vi "GetDeviceTransactions.vi"() -> ()   [LabVIEW 2014]
uses:
  USBAnalyzerEllisysDll/Debug/USBAnalyzerEllisysDll.dll
panel:
  out "Dev":i32[](array[numeric])
  out "devices 2":i32[](array[numeric])
  out "transactions":u64[](array[numeric])
  out "size":i32
  out "Percent %":dbl[](array[numeric]) format="%.2f"
  out "Pie Chart":picture
  out "Colors 2":u32[](array[colorbox])=[11796480, 37103, 40712, 16770816, 11796658, 4210752]
  in  "Colors":u32[](array[colorbox])=[11796480, 37103, 40712, 16770816, 11796658, 4210752]
  out "return type":i32
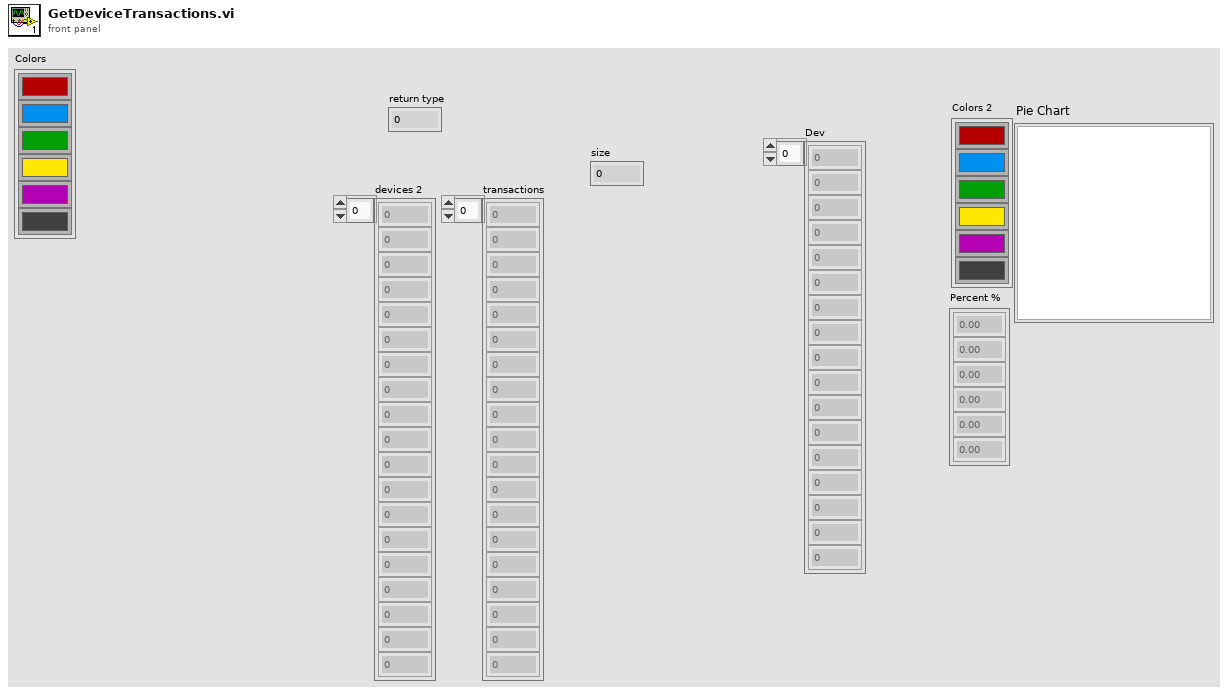
[diagram p1: front panel]
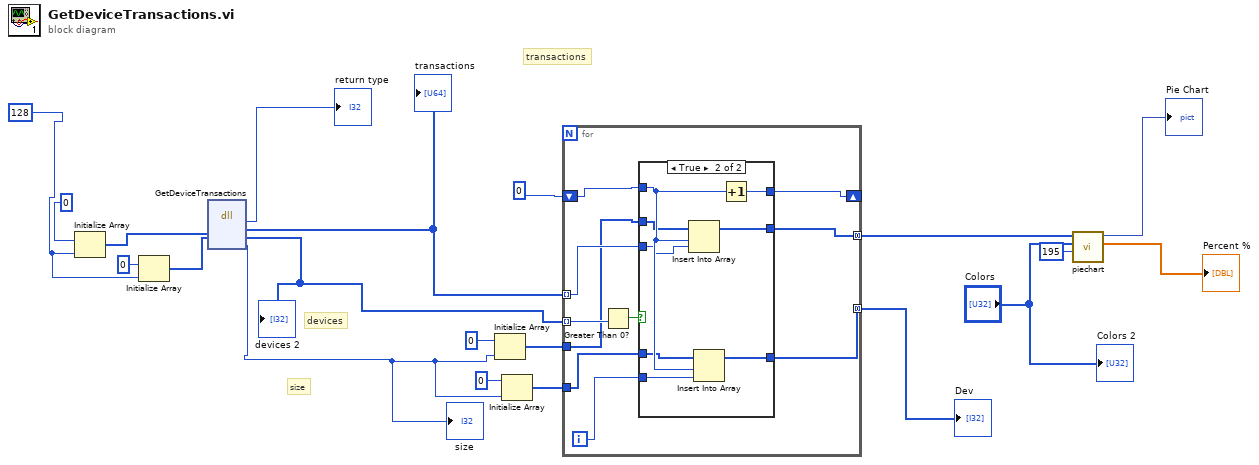
[diagram p0: block diagram]
diagram:
  w16 = 128
  # "size"
  # "transactions"
  # "devices"
  n1 = Initialize Array(u64 0 ("element"), w16) -> (w20:u64[])
  n2 = Initialize Array(0 ("element"), w16) -> (w18:i32[])
  n3 = dll-call lib="PTH2labs CUsersMichał\tDocumentsEllisysAnalyzerUSBAnalyzerEllisysDllDebugUSBAnalyzerEllisysDll.dll" fn="GetDeviceTransactions"("transactions"=w20, "devices"=w18) -> ("return type"=→"return type":i32, "transactions"=w3:u64[], "devices"=w4:i32[], "size"=w9:i32)  [unwired: 4 in, 2 out]
  "size" <- w9
  "transactions" <- w3
  "devices 2" <- w4
  n4 = Initialize Array(u64 0, w9) -> (w6:u64[])
  n5 = Initialize Array(0, w9) -> (w5:i32[])
  n6 = for {
    shift-right: [w29] -> _
    shift-left: 0 -> [w30]
    tunnel: w6 -> [w24]
    tunnel: w5 -> [w25]
    tunnel: w4 -> [w26] mode=indexing
    tunnel: w3 -> [w27] mode=indexing
    tunnel: [w22] -> w2 mode=concatenating
    tunnel: [w23] -> w1 mode=concatenating
    i -> [w21]
    n7 = Greater Than 0?(x=w26) -> (x > 0?=w28:bool)
    n8 = case shown="True" w28 {
      tunnel: w30 -> [w31 w38]
      tunnel: [w31 w39] -> w29
      tunnel: w27 -> [_ w37]
      tunnel: w24 -> [_ w36]
      tunnel: w25 -> [_ w35]
      tunnel: w21 -> [_ w34]
      tunnel: [_ w33] -> w23
      tunnel: [_ w32] -> w22
      frame False {
      }
      frame True {
        n9 = Insert Into Array(array=w36, index=w38, new element=w37) -> (w33:u64[])
        n10 = Insert Into Array(array=w35, index=w38, new element=w34) -> (w32:i32[])
        n11 = Increment(x=w38) -> (x+1=w39:i32)
      }
    }
  }
  "Dev" <- w2
  n12 = call "piechart.vi"("Pie Chart Size"=i16 195, "Colors"="Colors", "Values"=w1) -> ("Percent %"=→"Percent %":dbl[], "Pie Chart"=→"Pie Chart":picture)  [unwired: 5 in]
  "Colors 2" <- "Colors"
